vi "Data averaging module.vi"(8 "error in (no error)":errorcluster, 11 "Logging queue element in":T2={"Imaging Protocol"=enum."Live Imaging", "Number of Trials"=0, "Frame Size"=512, "# Averaged frames"=0, "Dwell time (us)"=0.0, "Index of Z-plane"=0, "Timelapse?"=FALSE, "Logging process is active"=FALSE, "Speed logging enabled"=FALSE, "tdms file ref"=refnum, "path"=path "", "Trial Number"=0, "Expected # points acquired"=FALSE, "Manually stopped"=FALSE, "Last trial"=FALSE, "Ch0 data"=[], "Ch1 data"=[], "Ref Data"=[], "Ref Frame Time"=[], "Image Time"=[], "Continuous Time"=[], "Ref X Length"=0, "Ref Y Length"=0, "# Ref Averaged frames"=0, "Ref Dwell time (us)"=0.0, "Points acquired"={"Ch0 last trial"=0, "Ch1 last trial"=0, "All trials"=0}, "HW Timings File"=refnum} {"Ref Dwell time (us)" format="%#.6g"; "Frame Size" items=["100X100"=100, "128X128"=128, "200X200"=200, "256X256"=256, "512X512"=512, "1024x1024"=1024, "2048x2048"=2048]; "Dwell time (us)" format="%#.6g"}) -> (0 "error out":errorcluster, 1 "Ref Frame completed/generate image":bool, 2 "Standard Frame completed/generate image":bool, 3 "Single Frame Data":T1, 4 "Number of points in completed standard frame":i32, 5 "Movement Correction":bool, 6 "Number of points in completed Ref frame":i32)   [LabVIEW 2020]
uses:
  Typedefs/Logging queue element.ctl
  Typedefs/Imaging Protocols enum.ctl
  Typedefs/Frame Size.ctl
  Typedefs/Acquired points count.ctl
  Typedefs/Frame data dual cluster.ctl
panel:
  # "SUBROUTINE VI"
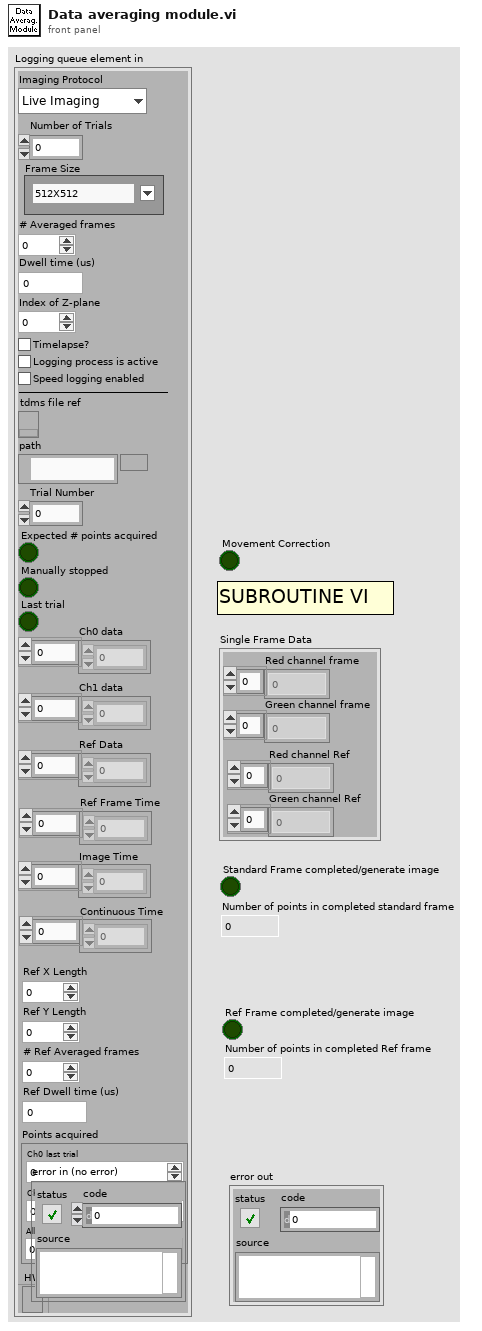
[diagram p1: front panel]
types:
  T1 = typedef "Frame data dual cluster.ctl" = cluster{"Red channel frame":dbl[], "Green channel frame":dbl[], "Red channel Ref":dbl[], "Green channel Ref":dbl[]}
  T2 = typedef "Logging queue element.ctl" = cluster{"Imaging Protocol":T3, "Number of Trials":u16, "Frame Size":T4, "# Averaged frames":u16, "Dwell time (us)":dbl, "Index of Z-plane":i32, "Timelapse?":bool, "Logging process is active":bool, "Speed logging enabled":bool, "tdms file ref":refnum<k34>, "path":path, "Trial Number":i32, "Expected # points acquired":bool, "Manually stopped":bool, "Last trial":bool, "Ch0 data":u32[], "Ch1 data":u32[], "Ref Data":u32[], "Ref Frame Time":u64[], "Image Time":u64[], "Continuous Time":u64[], "Ref X Length":u16, "Ref Y Length":u16, "# Ref Averaged frames":u16, "Ref Dwell time (us)":dbl, "Points acquired":T5, "HW Timings File":refnum<file>}
  T3 = typedef "Imaging Protocols enum.ctl" = enum16{"AOL Z-Stack", "Motor Z Stack", "Functional Acquisition", "Single Plane Acquisition", "Volume Acquisition", "Live Imaging", "Live Plane Imaging", "Live Volume Imaging"}
  T4 = typedef "Frame Size.ctl" = u16
  T5 = typedef "Acquired points count.ctl" = cluster{"Ch0 last trial":u64, "Ch1 last trial":u64, "All trials":u64}
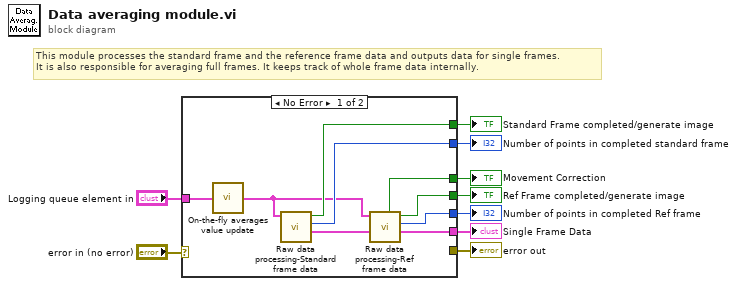
[diagram p0: block diagram]
diagram:
  # "This module processes the standard frame and the reference frame data and outputs data for single frames.\nIt is also responsible for averaging full frames. It keeps track of whole frame data internally."
  n1 = case shown="No Error" "error in (no error)" {
    selector: "error in (no error)" -> [_ w19]
    tunnel: "Logging queue element in" -> [w18 _]
    tunnel: [w16 _] -> w9
    tunnel: [_ w19] -> w7
    tunnel: [w14 _] -> w5
    tunnel: [w13 _] -> w4
    tunnel: [w17 _] -> w3
    tunnel: [w11 _] -> w2
    tunnel: [w10 _] -> w1
    frame No Error {
      n2 = call "On-the-fly averages value update.vi"("Logging queue element in"=w18) -> ("Logging queue element"=w12:T2)
      n3 = call "Raw data processing-Standard frame data.vi"("Logging queue element"=w12) -> ("Single Frame Data"=w15:T1, "Number of points in completed standard frame"=w17:i32, "Frame completed/generate image"=w16:bool)  [unwired: 8 in]
      n4 = call "Raw data processing-Ref frame data.vi"("Frame Data in"=w15, "Logging queue element"=w12) -> ("Frame Data"=w13:T1, "Number of points in completed Ref frame"=w11:i32, "Ref Frame completed/generate image"=w14:bool, "Movement Correction"=w10:bool)  [unwired: 6 in]
    }
    frame Error {
    }
  }
  "error out" <- w7
  "Standard Frame completed/generate image" <- w9
  "Number of points in completed standard frame" <- w3
  "Single Frame Data" <- w4
  "Ref Frame completed/generate image" <- w5
  "Number of points in completed Ref frame" <- w2
  "Movement Correction" <- w1
